vi "Timestamp to Posix String.vi"(11 "time stamp":timestamp) -> (3 "posix time string":string)   [LabVIEW 2018, in "Asset.lvclass"]
uses:
  Asset/Asset.lvclass
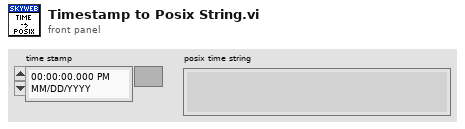
[diagram p1: front panel]
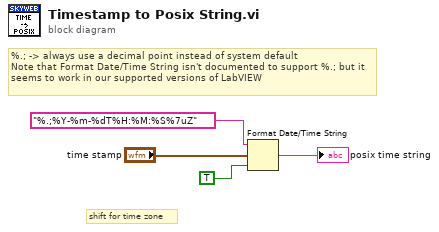
[diagram p0: block diagram]
diagram:
  # "%.; -> always use a decimal point instead of system default\nNote that Format Date/Time String isn't documented to support %.; but it seems to work in our supported versions of LabVIEW"
  # "shift for time zone"
  n1 = Format Date/Time String(time format string (%c)="%.;%Y-%m-%dT%H:%M:%S%7uZ", seconds (now)="time stamp", UTC format=TRUE) -> (date/time string=→"posix time string":string)
